vi "Update finished by name.vi"(8 "error in (no error)":errorcluster, 9 "Finished":bool, 10 "Name":string, 11 "Schedule in":refnum<class "Schedule.lvclass">) -> (0 "error out":errorcluster, 3 "Schedule out":refnum<class "Schedule.lvclass">)   [LabVIEW 2015, in "Schedule.lvclass"]
uses:
  Schedule.lvclass
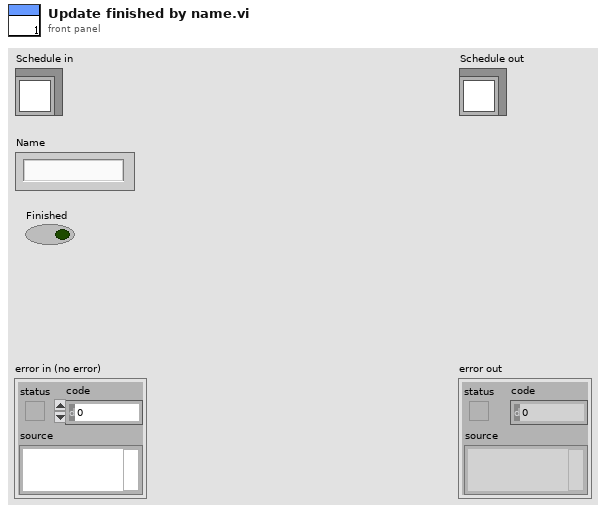
[diagram p1: front panel]
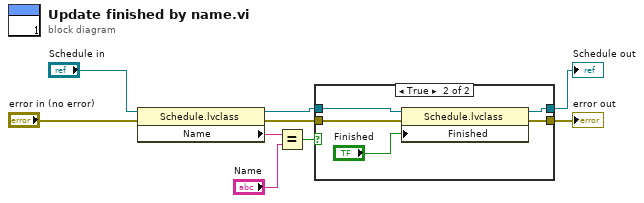
[diagram p0: block diagram]
diagram:
  n1 = property class="Schedule.lvclass"(reference="Schedule in", error in="error in (no error)") -> (reference out=w5:refnum<class "Schedule.lvclass">, error out=w4:errorcluster, "Name"=w8:string)
  n2 = Equal?(x=w8, y="Name") -> (x = y?=w6:bool)
  n3 = case shown="True" w6 {
    tunnel: w5 -> [w11 w16]
    tunnel: w4 -> [w10 w15]
    tunnel: [w11 w14] -> w3
    tunnel: [w10 w12] -> w2
    frame False {
    }
    frame True {
      n4 = property class="Schedule.lvclass"(reference=w16, error in=w15, "Finished"="Finished") -> (reference out=w14:refnum<class "Schedule.lvclass">, error out=w12:errorcluster)
    }
  }
  "error out" <- w2
  "Schedule out" <- w3
